vi "Write setup configuration.vi"(8 "error in (no error)":errorcluster, 11 "Channel in":refnum<class "SPARC4_Channel.lvclass">) -> (0 "error out":errorcluster, 3 "Channel out":refnum<class "SPARC4_Channel.lvclass">)   [LabVIEW 2018, in "SPARC4_Channel.lvclass"]
uses:
  SPARC4_Channel.lvclass
  SPARC4_Channel.lvclass/SPARC4_Channel.ctl
  Sim_CCD/Sim_CCD.lvclass/Sim_CCD.ctl
  Sim_Ixon_Ultra/Sim_Ixon_Ultra.lvclass
  C:/Users/Denis/Desktop/S4ACS/S4ACS/Sim_CCD/Sim_CCD.lvclass
  Sim_CCD/Sim_CCD.lvclass
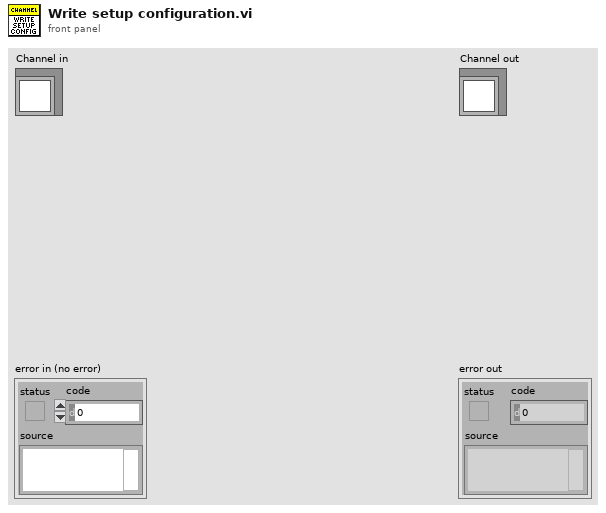
[diagram p1: front panel]
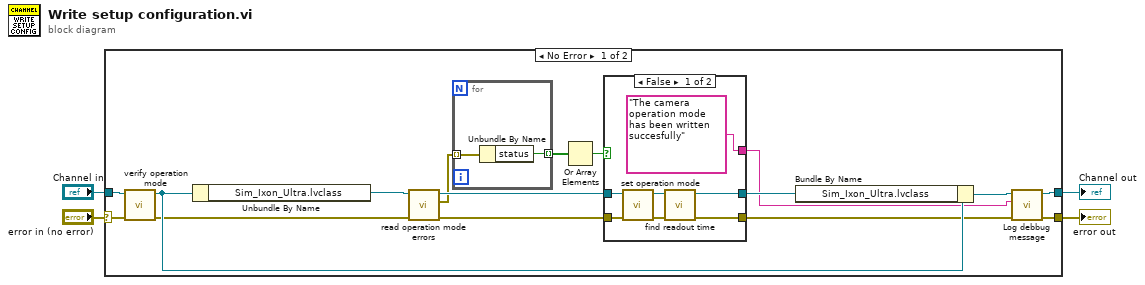
[diagram p0: block diagram]
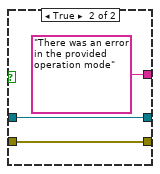
[diagram p2: hidden frame]
diagram:
  n1 = case shown="No Error" "error in (no error)" {
    selector: "error in (no error)" -> [w18 w34]
    tunnel: [w8 w34] -> w3
    tunnel: [w9 w33] -> w1
    tunnel: "Channel in" -> [w19 w33]
    frame No Error {
      n2 = call "verify operation mode.vi"("error in (no error)"=w18, "Channel in"=w19) -> ("error out"=w15:errorcluster, "Channel out"=w17:refnum<class "SPARC4_Channel.lvclass">)  [unwired: 8 in]
      n3 = Unbundle By Name(w17) -> ("Sim_Ixon_Ultra.lvclass"=w16:refnum<class "Sim_Ixon_Ultra.lvclass">)
      n4 = call "read operation mode errors.vi"("error in (no error)"=w15, "Simulated_CCD_Camera in"=w16) -> ("error out"=w14:errorcluster, "WRITE SETUP errors"=w12:errorcluster[], "Simulated_CCD_Camera out"=w13:refnum<class "Sim_Ixon_Ultra.lvclass">)  [unwired: 7 in]
      n5 = for {
        tunnel: w12 -> [w22] mode=indexing
        tunnel: [w21] -> w11 mode=indexing
        n6 = Unbundle By Name(w22) -> ("status"=w21:bool)
      }
      n7 = Or Array Elements(Boolean array=w11) -> (logical OR=w10:bool)
      n8 = case shown="False" w10 {
        tunnel: w13 -> [w29 w32]
        tunnel: w14 -> [w28 w31]
        tunnel: [w26 w31] -> w7
        tunnel: [w25 w32] -> w20
        tunnel: ["The camera operation mode has been written succesfully" ("String") "There was an error in the provided operation mode" ("String")] -> w5
        frame False {
          n9 = call-dynamic "set operation mode.vi"("error in (no error)"=w28, "CCDCamera in"=w29) -> ("error out"=w27:errorcluster, "CCDCamera out"=w24:refnum<class "Sim_Ixon_Ultra.lvclass">)  [unwired: 8 in]
          n10 = call-dynamic "find readout time.vi"("error in (no error)"=w27, "Simulated_CCD_Camera in"=w24) -> ("error out"=w26:errorcluster, "Simulated_CCD_Camera out"=w25:refnum<class "Sim_Ixon_Ultra.lvclass">)  [unwired: 8 in]
        }
        frame True {
        }
      }
      n11 = Bundle By Name(cluster=w17, "Sim_Ixon_Ultra.lvclass"=w20) -> (w6:refnum<class "SPARC4_Channel.lvclass">)
      n12 = call "Log debbug message.vi"("error in (no error)"=w7, "String"=w5, "Channel in"=w6) -> ("error out"=w8:errorcluster, "Channel out"=w9:refnum<class "SPARC4_Channel.lvclass">)  [unwired: 7 in]
    }
    frame Error {
    }
  }
  "error out" <- w3
  "Channel out" <- w1
